vi "2D array-index diagonal elements-NW to SE.vi"(7 "Diagonal direction":T1, 8 "error in (no error)":errorcluster, 9 "no. of elements (dflt=4)":i32=4, 10 "index of first element":cluster{"i":u32, "j":u32}, 11 "2D array in":i32[][](array[numeric])=[[8, 2, 22, 97, 38, 15, 0, 40, 0, 75], [49, 49, 99, 40, 17, 81, 18, 57, 60, 87], [81, 49, 31, 73, 55, 79, 14, 29, 93, 71], [52, 70, 95, 23, 4, 60, 11, 42, 69, 24], [22, 31, 16, 71, 51, 67, 63, 89, 41, 92], [24, 47, 32, 60, 99, 3, 45, 2, 44, 75], [32, 98, 81, 28, 64, 23, 67, 10, 26, 38], [67, 26, 20, 68, 2, 62, 12, 20, 95, 63], [24, 55, 58, 5, 66, 73, 99, 26, 97, 17], [21, 36, 23, 9, 75, 0, 76, 44, 20, 45]]) -> (0 "error out":errorcluster, 3 "Diagonal elements out":i32[](array[numeric])=[8, 2, 22, 97, 38, 15, 0, 40, 0, 75])   [LabVIEW 2021, in "Numeric Utilities.lvlib"]
uses:
  Numeric Utilities.lvlib
  diagonal direction.ctl
panel:
  out "T = all diagonal elements requested are inside the 2D array":bool
  out "no. of columns":i32
  out "no. of rows":i32
  out "T = first element is inside the 2D array":bool
  # "Development\ncontrols/indicators useful for development and testing, but which are not outputs of the VI"
  # "Input\nInputs to the VI"
  # "Output\nOutputs of the VI"
  # "Description\n\nBlank VI with error handling case. \n\nSummarize the use of this VI in this space."
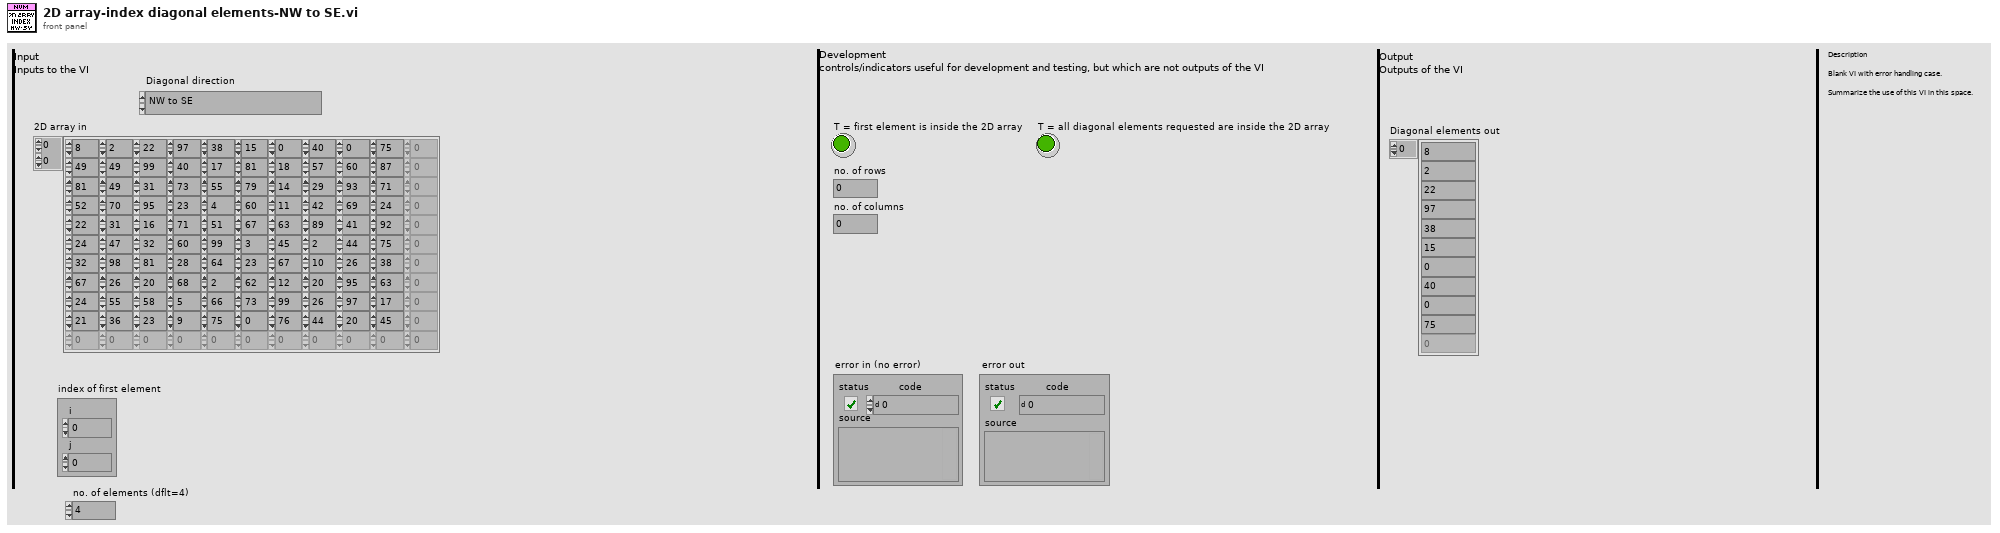
[diagram p1: front panel]
types:
  T1 = typedef "Numeric Utilities.lvlib/diagonal direction.ctl" = enum16{"NW to SE", "SE to NW", "NE to SW", "SW to NE"}
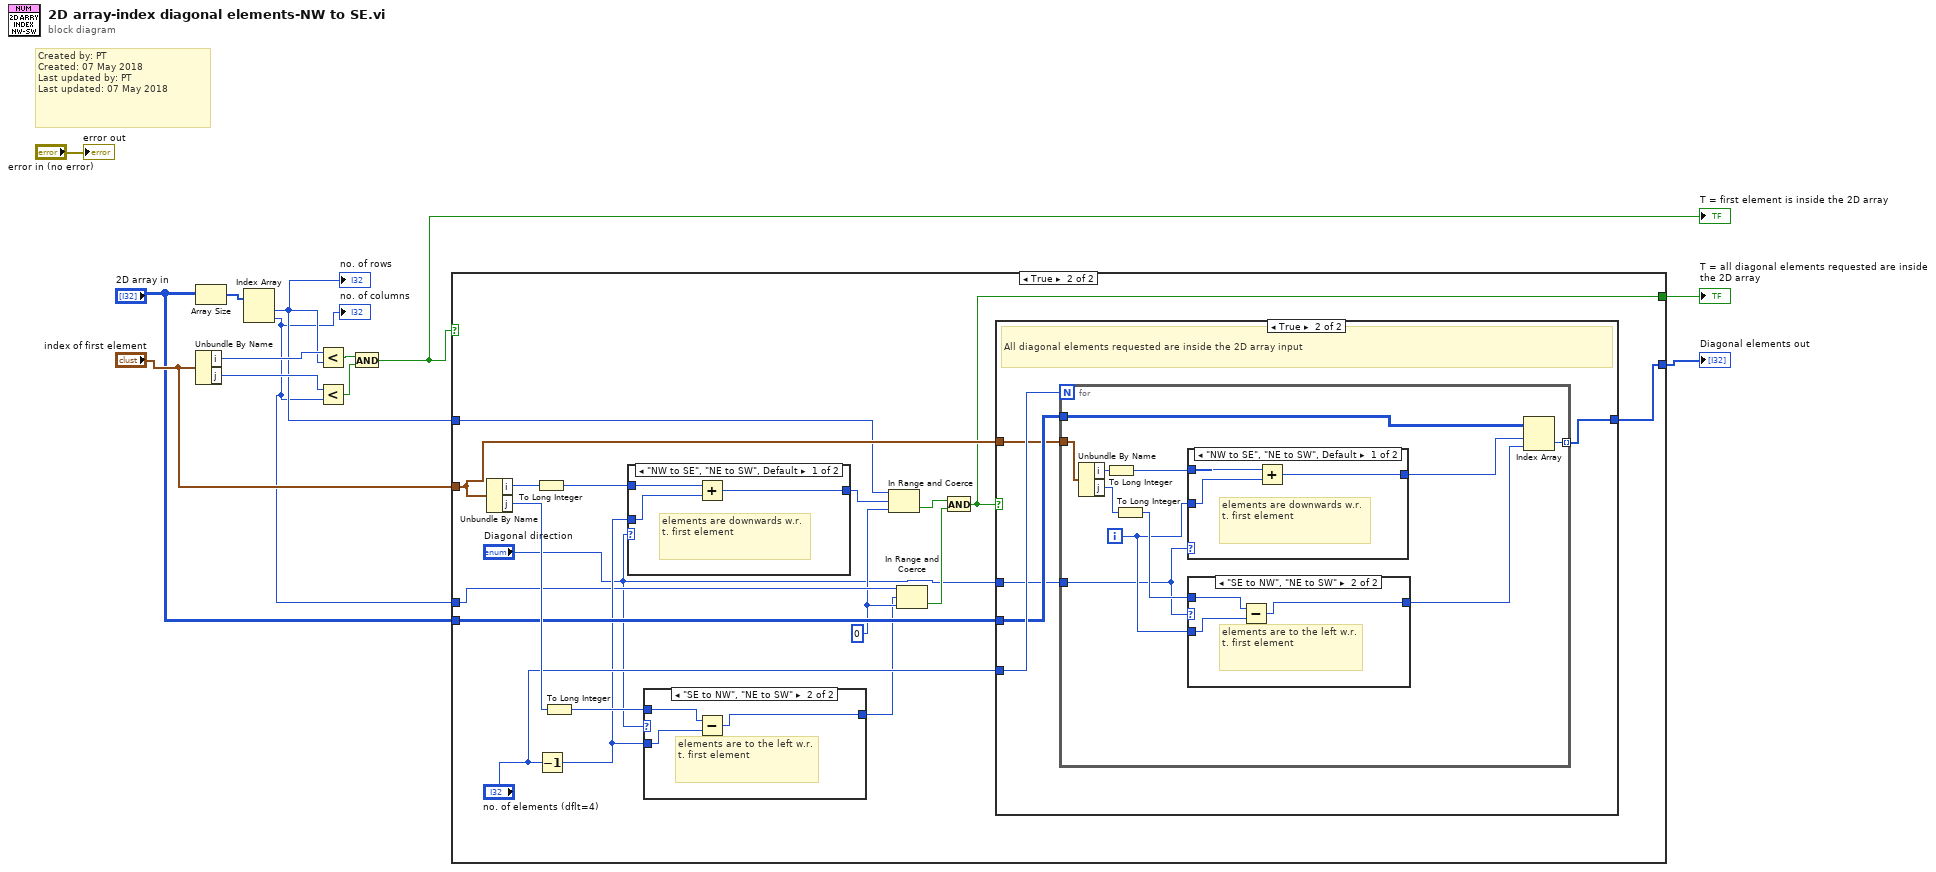
[diagram p0: block diagram]
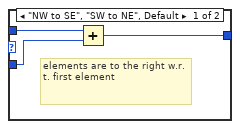
[diagram p3: hidden frame]
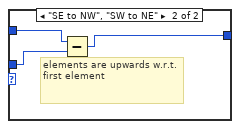
[diagram p4: hidden frame]
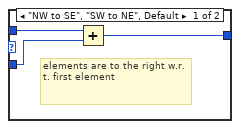
[diagram p6: hidden frame]
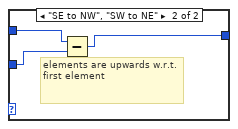
[diagram p7: hidden frame]
diagram:
  # "Created by: PT\nCreated: 07 May 2018\nLast updated by: PT\nLast updated: 07 May 2018"
  n1 = Array Size(array="2D array in") -> (size(s)=w12:i32[])
  n2 = Unbundle By Name("index of first element") -> ("i"=w11:u32, "j"=w10:u32)
  n3 = Index Array(array=w12) -> (element #1=w6:i32, element #2=w4:i32)  [unwired: 2 in]
  "no. of rows" <- w6
  "no. of columns" <- w4
  n4 = Less?(x=w11, y=w6) -> (x < y?=w9:bool)
  n5 = Less?(x=w10, y=w4) -> (x < y?=w8:bool)
  n6 = And(x=w9, y=w8) -> (x .and. y?=w7:bool)
  "T = first element is inside the 2D array" <- w7
  n7 = case shown="True" w7 {
    tunnel: [_ w26] -> w1
    tunnel: w6 -> [_ w21]
    tunnel: "index of first element" -> [_ w24]
    tunnel: w4 -> [_ w17]
    tunnel: "2D array in" -> [_ w25]
    tunnel: [_ w22] -> w2
    frame False {
    }
    frame True {
      w16 = 0 ("lower limit")
      n8 = Unbundle By Name(w24) -> ("i"=w31:u32, "j"=w28:u32)
      n9 = To Long Integer(number=w31) -> (32bit integer=w30:i32)
      n10 = Decrement(x="no. of elements (dflt=4)") -> (x-1=w18:i32)
      n11 = To Long Integer(number=w28) -> (32bit integer=w19:i32)
      n12 = case shown="\"NW to SE\", \"NE to SW\", Default" "Diagonal direction" {
        tunnel: [w40 w41] -> w20
        tunnel: w30 -> [w39 w43]
        tunnel: w18 -> [w38 w42]
        frame "NW to SE", "NE to SW", Default {
          # "elements are downwards w.r.t. first element"
          n13 = Add(x=w39, y=w38) -> (x+y=w40:i32)
        }
        frame "SE to NW", "SW to NE" {
          # "elements are upwards w.r.t. first element"
          n14 = Subtract(x=w43, y=w42) -> (x-y=w41:i32)
        }
      }
      n15 = case shown="\"SE to NW\", \"NE to SW\"" "Diagonal direction" {
        tunnel: [w34 w35] -> w15
        tunnel: w19 -> [w33 w37]
        tunnel: w18 -> [w32 w36]
        frame "NW to SE", "SW to NE", Default {
          # "elements are to the right w.r.t. first element"
          n16 = Add(x=w33, y=w32) -> (x+y=w34:i32)
        }
        frame "SE to NW", "NE to SW" {
          # "elements are to the left w.r.t. first element"
          n17 = Subtract(x=w37, y=w36) -> (x-y=w35:i32)
        }
      }
      n18 = In Range and Coerce(upper limit=w21, x=w20, lower limit=w16) -> (In Range?=w29:bool)  [unwired: 1 out]
      n19 = In Range and Coerce(upper limit=w17, x=w15, lower limit=w16) -> (In Range?=w27:bool)  [unwired: 1 out]
      n20 = And(x=w29, y=w27) -> (x .and. y?=w22:bool)
      n21 = case shown="True" w22 {
        tunnel: [_ w45] -> w26
        tunnel: "no. of elements (dflt=4)" -> [_ w48]
        tunnel: w25 -> [_ w47]
        tunnel: w24 -> [_ w46]
        tunnel: "Diagonal direction" -> [_ w44]
        frame False {
          # "Some diagonal requested elements are outside of the bounds of the 2D array input.\nDesign decision: return empty array when this happens."
        }
        frame True {
          # "All diagonal elements requested are inside the 2D array input"
          n22 = for {
            N: w48 -> [_]
            tunnel: w47 -> [w59]
            tunnel: w46 -> [w58]
            tunnel: [w55] -> w45 mode=indexing
            tunnel: w44 -> [w50]
            i -> [w51]
            n23 = Unbundle By Name(w58) -> ("i"=w57:u32, "j"=w56:u32)
            n24 = To Long Integer(number=w57) -> (32bit integer=w54:i32)
            n25 = To Long Integer(number=w56) -> (32bit integer=w52:i32)
            n26 = case shown="\"NW to SE\", \"NE to SW\", Default" w50 {
              tunnel: [w68 w69] -> w53
              tunnel: w54 -> [w67 w71]
              tunnel: w51 -> [w66 w70]
              frame "NW to SE", "NE to SW", Default {
                # "elements are downwards w.r.t. first element"
                n27 = Add(x=w67, y=w66) -> (x+y=w68:i32)
              }
              frame "SE to NW", "SW to NE" {
                # "elements are upwards w.r.t. first element"
                n28 = Subtract(x=w71, y=w70) -> (x-y=w69:i32)
              }
            }
            n29 = case shown="\"SE to NW\", \"NE to SW\"" w50 {
              tunnel: [w62 w63] -> w49
              tunnel: w52 -> [w61 w65]
              tunnel: w51 -> [w60 w64]
              frame "NW to SE", "SW to NE", Default {
                # "elements are to the right w.r.t. first element"
                n30 = Add(x=w61, y=w60) -> (x+y=w62:i32)
              }
              frame "SE to NW", "NE to SW" {
                # "elements are to the left w.r.t. first element"
                n31 = Subtract(x=w65, y=w64) -> (x-y=w63:i32)
              }
            }
            n32 = Index Array(array=w59, index (row)=w53, index (col)=w49) -> (element=w55:i32)
          }
        }
      }
    }
  }
  "Diagonal elements out" <- w1
  "T = all diagonal elements requested are inside the 2D array" <- w2
  "error out" <- "error in (no error)"
